vi "mxwScript_API_SetVal_NamedXNodeState.vi"(8 "error in (no error)":errorcluster, 10 "XNode state":T2, 11 "XNode name":string) -> (0 "error out":errorcluster, 3 "parameter":T1)   [LabVIEW 2017]
uses:
  codeGenAPISupport.llb/cgAPI_mxwScript_XNodeState.ctl
  codeGenAPISupport.llb/cgAPI_mxwScript_VersionInfo.ctl
  codeGenAPISupport.llb/cgAPI_mxwScript_Parameter.ctl
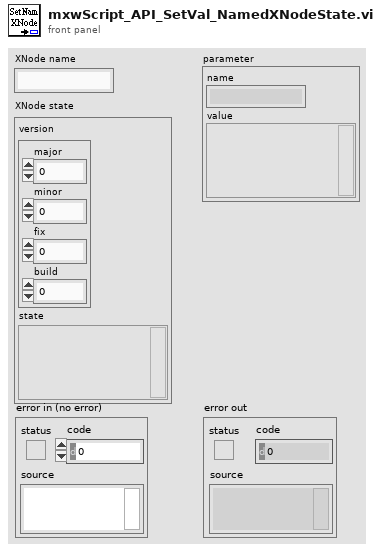
[diagram p1: front panel]
types:
  T1 = typedef "cgAPI_mxwScript_Parameter.ctl" = cluster{"name":string, "value":variant}
  T2 = typedef "cgAPI_mxwScript_XNodeState.ctl" = cluster{"version":T3, "state":variant}
  T3 = typedef "cgAPI_mxwScript_VersionInfo.ctl" = cluster{"major":u16, "minor":u16, "fix":u16, "build":u16}
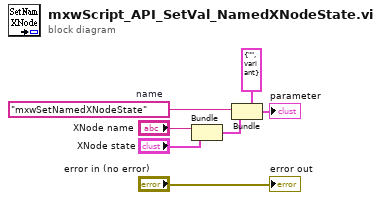
[diagram p0: block diagram]
diagram:
  w4 = "mxwSetNamedXNodeState"  # name
  n1 = Bundle("XNode name"="XNode name", "XNode state"="XNode state") -> (w1:cluster{"XNode name":string, "XNode state":T2})  [unwired: 1 out]
  n2 = Bundle(cluster=T1 {"name"="", "value"=variant} ("parameter"), "name"=w4, "value"=w1) -> (→"parameter":T1)
  "error out" <- "error in (no error)"
